vi "GrGFASTAcquireDSO1004.vi"() -> ()   [LabVIEW 2011]
doc: "This example shows how to configure multiple channels and acquire waveforms from multiple channels."
uses:
  <instrlib>/Agilent DSO1000 Series/Public/Data/Read Waveform (Multiple).vi
  <vilib>/Waveform/WDTFileIO.llb/Export Waveforms To Spreadsheet File (1D).vi
  <instrlib>/Agilent DSO1000 Series/Agilent DSO1000 Series.lvlib
panel:
  in  "File Path Control":path=path "E:/Documents/MSU/Research/Measurement/PlateProperties/MulticycleSignal/F100kD4cm.txt"
  in  "stop":bool
  in  "Maximum Time (10000 ms)":u32=10000
  out "Waveform Data":waveform(dbl)[](graph)=[{"t0"=timestamp(-5.9999998484050465e-05 s since 1904-01-01), "dt"=2e-07, "Y"=[0.0, 0.4, 0.0, 0.4, 0.0, 0.4, 0.0, 0.4, 0.4, 0.0, 0.4, 0.0, 0.0, 0.4, 0.4, 0.0, 0.4, 0.0, 0.4, 0.0, 0.0, 0.4, 0.4, 0.0, 0.0, 0.4, 0.0, 0.4, 0.0, 0.4, 0.4, 0.0, 0.0, 0.4, 0.4, 0.0, 0.4, 0.0, 0.0, 0.4, 0.4, 0.0, 0.0, 0.4, 0.4, 0.0, 0.4, 0.0, 0.4, 0.0, 0.0, 0.4, 0.0, 0.4, 0.0, 0.4, 0.0, 0.4, 0.0, 0.4, 0.4, 0.0, 0.0, 0.4, 0.0, 0.4, 0.0, 0.4, 0.0, 0.0, 0.4, 0.0, 0.0, 0.4, 0.0, 0.4, 0.0, 0.4, 0.0, 0.4, 0.0, 0.4, 0.0, 0.4, 0.4, 0.0, 0.0, 0.4, 0.4, 0.0, 0.0, 0.0, 0.0, 0.4, 0.0, 0.4, 0.4, 0.0, 0.0, 0.4, 0.4, 0.0, 0.0, 0.4, 0.0, 0.4, 0.0, 0.4, 0.0, 0.4, 0.0, 0.4, 0.0, 0.4, 0.0, 0.4, 0.0, 0.4, 0.4, 0.0, 0.0, 0.4, 0.4, 0.0, 0.0, 0.4, 0.4, 0.0, 0.0, 0.4, 0.0, 0.4, 0.0, 0.4, 0.4, 0.0, 0.0, 0.4, 0.4, 0.0, 0.0, 0.4, 0.0, 0.4, 0.0, 0.4, 0.0, 0.4, 0.0, 0.4, 0.4, 0.0, 0.4, 0.0, 0.4, 0.0, 0.0, 0.4, 0.0, 0.4, 0.4, 0.0, 0.0, 0.4, 0.0, 0.4, 0.0, 0.4, 0.0, 0.4, 0.0, 0.4, 0.0, 0.4, 0.4, 0.0, 0.4, 0.0, 0.4, 0.0, 0.4, 0.0, 0.4, 0.0, 0.4, 0.0, 0.0, 0.4, 0.0, 0.4, 0.4, 0.0, 0.0, 0.4, 0.4, 0.0, 0.0, 0.4, 0.0, 0.4, 0.0, 0.4, 0.0, 0.4, 0.0, 0.4, 0.0, 0.4, 0.0, 0.4, 0.0, 0.4, 0.0, 0.4, 0.4, 0.0, 0.4, 0.0, 0.0, 0.4, 0.0, 0.4, 0.0, 0.4, 0.0, 0.4, 0.0, 0.4, 0.0, 0.4, 0.0, 0.4, 0.0, 0.4, 0.0, 0.4, 0.0, 0.4, 0.4, 0.0, 0.0, 0.4, 0.4, 0.0, 0.4, 0.0, 0.4, 0.0, 0.4, 0.0, 0.4, 0.0, 0.4, 0.0, 0.0, 0.4, 0.0, 0.4, 0.4, 0.0, 0.0, 0.4, 0.4, 0.4, 0.4, 0.4, 0.4, 0.4, 0.4, 0.0, 0.0, 0.0, 0.0, -0.4, -0.4, 0.0, 0.0, 0.0, 0.0, 0.4, 0.4, 1.2000000000000002, 1.6, 1.2000000000000002, 1.6, 1.6, 1.6, 1.2000000000000002, 0.8, 0.0, -0.4, -1.2000000000000002, -1.6, -2.8000000000000003, -2.8000000000000003, -2.4000000000000004, -2.4000000000000004, -1.2000000000000002, -0.8, 1.2000000000000002, 1.6, 3.6, 3.6, 4.800000000000001, 5.2, 4.4, 4.4, 2.4000000000000004, 2.0, -0.8, -1.2000000000000002, -4.0, -4.4, -6.0, -6.0, -5.6000000000000005, -5.6000000000000005, -2.8000000000000003, -2.4000000000000004, 1.6, 2.0, 5.2, 6.0, 7.2, 7.2, 6.4, 6.0, 3.2, 3.2, -0.8, -1.2000000000000002, -4.4, -4.800000000000001, -6.0, -6.0, -5.2, -5.2, -2.4000000000000004, -2.4000000000000004, 1.2000000000000002, 1.6, 4.0, 4.0, 4.800000000000001, 4.800000000000001, 4.4, 4.4, 2.4000000000000004, 2.0, 0.0, -0.4, -2.0, -2.0, -2.8000000000000003, -2.8000000000000003, -2.0, -2.0, -0.8, -0.8, 0.4, 0.4, 1.6, 1.6, 1.6, 1.6, 1.6, 1.6, 0.8, 0.8, 0.0, 0.0, 0.0, 0.0, -0.4, 0.0, -0.4, 0.0, 0.0, 0.0, 0.0, 0.0, 0.4, 0.4, 0.4, 0.4, 0.4, 0.4, 0.0, 0.4, 0.0, 0.0, 0.4, 0.0, 0.0, 0.0, 0.0, 0.0, 0.0, 0.0, 0.4, 0.0, 0.4, 0.0, 0.4, 0.4, 0.0, 0.0, 0.4, 0.0, 0.4, 0.0, 0.4, 0.0, 0.4, 0.0, 0.4, 0.4, 0.0, 0.4, 0.0, 0.4, 0.0, 0.0, 0.4, 0.0, 0.4, 0.0, 0.4, 0.4, 0.0, 0.0, 0.4, 0.0, 0.4, 0.0, 0.4, 0.0, 0.4, 0.4, 0.0, 0.0, 0.4, 0.4, 0.0, 0.0, 0.4, 0.4, 0.0, 0.0, 0.4, 0.0, 0.4, 0.0, 0.4, 0.0, 0.4, 0.0, 0.4, 0.0, 0.4, 0.4, 0.0, 0.0, 0.4, 0.0, 0.4, 0.0, 0.4, 0.0, 0.4, 0.0, 0.4, 0.4, 0.0, 0.4, 0.0, 0.4, 0.0, 0.4, 0.0, 0.0, 0.4, 0.0, 0.4, 0.0, 0.4, 0.0, 0.4, 0.0, 0.4, 0.0, 0.4, 0.0, 0.4, 0.4, 0.0, 0.0, 0.4, 0.4, 0.0, 0.4, 0.0, 0.0, 0.4, 0.0, 0.0, 0.4, 0.0, 0.4, 0.0, 0.0, 0.4, 0.0, 0.4, 0.0, 0.4, 0.4, 0.0, 0.0, 0.0, 0.0, 0.4, 0.0, 0.4, 0.0, 0.4, 0.4, 0.0, 0.0, 0.4, 0.4, 0.0, 0.4, 0.0, 0.0, 0.4, 0.0, 0.4, 0.4, 0.0, 0.0, 0.0, 0.4, 0.0, 0.0, 0.4, 0.0, 0.4, 0.0, 0.4, 0.0, 0.4, 0.0, 0.4, 0.0, 0.4, 0.0, 0.4, 0.4, 0.0, 0.0, 0.4, 0.0, 0.0, 0.4, 0.0, 0.0, 0.4, 0.4, 0.0, 0.0, 0.0, 0.4, 0.0, 0.0, 0.4, 0.0, 0.4, 0.0, 0.4, 0.0, 0.4, 0.0, 0.4, 0.0, 0.4, 0.0, 0.0, 0.0, 0.4, 0.4, 0.0, 0.0, 0.4, 0.0, 0.4, 0.4, 0.0, 0.0, 0.4]}, {"t0"=timestamp(-5.9999998484050465e-05 s since 1904-01-01), "dt"=2e-07, "Y"=[0.004, 0.0, 0.0, 0.004, 0.0, 0.004, 0.0, 0.004, 0.004, 0.0, 0.004, 0.0, 0.0, 0.004, 0.0, 0.004, 0.0, 0.004, 0.004, 0.0, 0.0, 0.004, 0.004, 0.0, 0.0, 0.004, 0.004, 0.0, 0.004, 0.0, 0.004, 0.0, 0.004, 0.0, 0.0, 0.004, 0.0, 0.004, 0.0, 0.004, 0.0, 0.004, 0.004, 0.0, 0.0, 0.004, 0.0, 0.004, 0.0, 0.004, 0.004, 0.0, 0.0, 0.004, 0.0, 0.004, 0.0, 0.004, 0.0, 0.004, 0.0, 0.004, 0.0, 0.004, 0.0, 0.004, 0.0, 0.004, 0.004, 0.0, 0.004, 0.0, 0.0, 0.004, 0.0, 0.004, 0.0, 0.004, 0.004, 0.0, 0.0, 0.004, 0.0, 0.004, 0.0, 0.004, 0.0, 0.004, 0.0, 0.0, 0.0, 0.004, 0.0, 0.004, 0.004, 0.0, 0.0, 0.004, 0.0, 0.0, 0.0, 0.004, 0.004, 0.0, 0.0, 0.004, 0.0, 0.004, 0.0, 0.004, 0.0, 0.004, 0.0, 0.004, 0.0, 0.004, 0.004, 0.0, 0.004, 0.0, 0.0, 0.004, 0.0, 0.004, 0.0, 0.004, 0.0, 0.0, 0.0, 0.004, 0.004, 0.0, 0.0, 0.004, 0.004, 0.0, 0.0, 0.004, 0.0, 0.004, 0.0, 0.004, 0.004, 0.0, 0.0, 0.004, 0.0, 0.004, 0.0, 0.004, 0.0, 0.004, 0.004, 0.0, 0.0, 0.004, 0.0, 0.004, 0.0, 0.004, 0.0, 0.004, 0.0, 0.004, 0.004, 0.0, 0.0, 0.004, 0.0, 0.004, 0.0, 0.004, 0.004, 0.0, 0.0, 0.004, 0.0, 0.004, 0.0, 0.004, 0.0, 0.004, 0.0, 0.004, 0.0, 0.004, 0.0, 0.004, 0.0, 0.004, 0.0, 0.0, 0.0, 0.004, 0.004, 0.0, 0.004, 0.0, 0.0, 0.004, 0.0, 0.004, 0.0, 0.004, 0.004, 0.0, 0.0, 0.004, 0.004, 0.0, 0.0, 0.004, 0.004, 0.0, 0.0, 0.004, 0.004, 0.0, 0.0, 0.004, 0.0, 0.004, 0.0, 0.004, 0.0, 0.004, 0.004, 0.0, 0.0, 0.0, 0.0, 0.004, 0.0, 0.004, 0.0, 0.004, 0.0, 0.004, 0.004, 0.0, 0.004, 0.0, 0.0, 0.004, 0.004, 0.0, 0.004, 0.0, 0.0, 0.004, 0.0, 0.004, 0.0, 0.004, 0.0, 0.004, 0.0, 0.004, 0.0, 0.004, 0.0, 0.004, 0.004, 0.0, 0.0, 0.004, 0.0, 0.004, 0.004, 0.0, 0.0, 0.004, 0.0, 0.004, 0.0, 0.004, 0.004, 0.0, 0.004, 0.0, 0.0, 0.004, 0.0, 0.004, 0.0, 0.004, 0.0, 0.004, 0.004, 0.0, 0.004, 0.0, 0.004, 0.0, 0.0, 0.004, 0.004, 0.0, 0.0, 0.004, 0.0, 0.004, 0.004, 0.0, 0.004, 0.0, 0.004, 0.0, 0.0, 0.004, 0.0, 0.004, 0.0, 0.004, 0.0, 0.004, 0.0, 0.004, 0.004, 0.0, 0.0, 0.004, 0.0, 0.004, 0.0, 0.004, 0.0, 0.004, 0.004, 0.0, 0.0, 0.004, 0.0, 0.004, 0.0, 0.004, 0.0, 0.004, 0.0, 0.004, 0.0, 0.004, 0.0, 0.004, 0.0, 0.004, 0.004, 0.0, 0.0, 0.004, 0.0, 0.004, 0.0, 0.004, 0.004, 0.0, 0.0, 0.004, 0.0, 0.004, 0.0, 0.004, 0.004, 0.0, 0.0, 0.004, 0.004, 0.0, 0.004, 0.0, 0.004, 0.0, 0.004, 0.0, 0.0, 0.004, 0.0, 0.004, 0.0, 0.004, 0.004, 0.0, 0.0, 0.004, 0.0, 0.004, 0.0, 0.004, 0.004, 0.0, 0.0, 0.004, 0.0, 0.004, 0.004, 0.0, 0.0, 0.004, 0.004, 0.0, 0.0, 0.004, 0.004, 0.0, 0.0, 0.0, 0.0, 0.004, 0.0, 0.004, 0.0, 0.0, 0.0, 0.004, 0.004, 0.0, 0.004, 0.0, 0.0, 0.004, 0.0, 0.004, 0.0, 0.004, 0.004, 0.0, 0.0, 0.004, 0.0, 0.004, 0.0, 0.004, 0.0, 0.004, 0.0, 0.0, 0.0, 0.004, 0.0, 0.004, 0.0, 0.004, 0.004, 0.0, 0.0, 0.004, 0.0, 0.004, 0.004, 0.0, 0.0, 0.0, 0.0, 0.0, 0.0, 0.004, 0.0, 0.004, 0.0, 0.004, 0.0, 0.004, 0.004, 0.0, 0.0, 0.004, 0.0, 0.004, 0.004, 0.0, 0.004, 0.0, 0.0, 0.004, 0.0, 0.004, 0.004, 0.0, 0.004, 0.0, 0.004, 0.0, 0.004, 0.0, 0.0, 0.004, 0.0, 0.004, 0.004, 0.0, 0.0, 0.004, 0.0, 0.004, 0.004, 0.0, 0.0, 0.004, 0.0, 0.0, 0.0, 0.004, 0.0, 0.004, 0.0, 0.004, 0.004, 0.0, 0.004, 0.0, 0.0, 0.004, 0.0, 0.004, 0.004, 0.0, 0.0, 0.004, 0.0, 0.004, 0.004, 0.0, 0.0, 0.0, 0.004, 0.0, 0.0, 0.004, 0.0, 0.004, 0.0, 0.004, 0.0, 0.004, 0.0, 0.0, 0.0, 0.004, 0.0, 0.004, 0.0, 0.004, 0.0, 0.004, 0.004, 0.0, 0.0, 0.004, 0.0, 0.004, 0.0, 0.004, 0.0, 0.004, 0.004, 0.0, 0.004, 0.0, 0.004, 0.0, 0.004, 0.0, 0.0, 0.0, 0.0, 0.004, 0.0, 0.004, 0.0, 0.004, 0.0, 0.004, 0.004, 0.0, 0.004, 0.0, 0.004, 0.0, 0.0, 0.004, 0.0, 0.004, 0.0, 0.004, 0.0, 0.004, 0.0, 0.004, 0.0, 0.004, 0.0, 0.004, 0.0, 0.004, 0.0, 0.004, 0.004, 0.0, 0.0, 0.004]}, {"t0"=timestamp(-5.9999998484050465e-05 s since 1904-01-01), "dt"=2e-07, "Y"=[0.0, 0.0, 0.0, 0.0, 0.0, 0.0, 0.0, 0.0, 0.0, 0.0, 0.0, 0.0, 0.0, 0.0, 0.0, 0.0, 0.0, 0.0, 0.0, 0.0, 0.0, 0.0, 0.0, 0.0, 0.0, 0.0, 0.0, 0.0, 0.0, 0.0, 0.0, 0.0, 0.0, 0.0, 0.0, 0.0, 0.0, 0.0, 0.0, 0.0, 0.0, 0.0, 0.0, 0.0, 0.0, 0.0, 0.0, 0.0, 0.0, 0.0, 0.0, 0.0, 0.0, 0.0, 0.0, 0.0, 0.0, 0.0, 0.0, 0.0, 0.0, 0.0, 0.0, 0.4, 0.0, 0.0, 0.0, 0.0, 0.0, 0.0, 0.0, 0.0, 0.0, 0.0, 0.0, 0.0, 0.0, 0.0, 0.0, 0.4, 0.0, 0.0, 0.0, 0.0, 0.0, 0.0, 0.0, 0.0, 0.0, 0.0, 0.0, 0.0, 0.0, 0.0, 0.0, 0.4, 0.0, 0.0, 0.0, 0.0, 0.0, 0.0, 0.0, 0.0, 0.0, 0.0, 0.0, 0.0, 0.0, 0.0, 0.0, 0.0, 0.0, 0.0, 0.0, 0.0, 0.0, 0.0, 0.0, 0.0, 0.0, 0.0, 0.0, 0.0, 0.0, 0.0, 0.0, 0.0, 0.0, 0.0, 0.0, 0.0, 0.0, 0.0, 0.0, 0.0, 0.0, 0.0, 0.0, 0.0, 0.0, 0.4, 0.0, 0.0, 0.0, 0.0, 0.0, 0.0, 0.0, 0.0, 0.0, 0.0, 0.0, 0.0, 0.0, 0.0, 0.0, 0.0, 0.0, 0.0, 0.0, 0.0, 0.0, 0.0, 0.0, 0.0, 0.0, 0.0, 0.0, 0.0, 0.0, 0.0, 0.0, 0.0, 0.0, 0.0, 0.0, 0.0, 0.0, 0.0, 0.0, 0.0, 0.0, 0.0, 0.0, 0.0, 0.0, 0.0, 0.0, 0.0, 0.0, 0.0, 0.0, 0.0, 0.0, 0.0, 0.0, 0.0, 0.0, 0.0, 0.0, 0.0, 0.0, 0.0, 0.0, 0.0, 0.0, 0.0, 0.0, 0.0, 0.0, 0.0, 0.0, 0.0, 0.0, 0.0, 0.0, 0.0, 0.0, 0.0, 0.0, 0.4, 0.0, 0.0, 0.0, 0.0, 0.0, 0.0, 0.0, 0.0, 0.0, 0.0, 0.0, 0.0, 0.0, 0.0, 0.0, 0.0, 0.0, 0.0, 0.0, 0.0, 0.0, 0.0, 0.0, 0.0, 0.0, 0.0, 0.0, 0.0, 0.0, 0.0, 0.0, 0.0, 0.0, 0.0, 0.0, 0.0, 0.0, 0.0, 0.0, 0.0, 0.0, 0.0, 0.0, 0.0, 0.0, 0.4, 0.0, 0.0, 0.0, 0.0, 0.0, 0.0, 0.0, 0.0, 0.0, 0.0, 0.0, 0.0, 0.0, 0.0, 0.0, 0.0, 0.0, 0.0, 0.0, 0.0, 0.0, 0.0, 0.0, 0.0, 0.0, 0.0, 0.0, 0.0, 0.0, 0.0, 0.0, 0.0, 0.0, 0.0, 0.0, 0.0, 0.0, 0.0, 0.0, 0.0, 0.0, 0.0, 0.0, 0.0, 0.0, 0.0, 0.0, 0.0, 0.0, 0.0, 0.0, 0.0, 0.0, 0.0, 0.0, 0.0, 0.0, 0.0, 0.0, 0.0, 0.0, 0.0, 0.0, 0.0, 0.0, 0.0, 0.0, 0.0, 0.0, 0.0, 0.0, 0.0, 0.0, 0.0, 0.0, 0.0, 0.0, 0.0, 0.0, 0.0, 0.0, 0.4, 0.0, 0.4, 0.0, 0.0, 0.0, 0.0, 0.0, 0.0, 0.0, 0.0, 0.0, 0.0, 0.0, 0.0, 0.0, 0.0, 0.0, 0.0, 0.0, 0.0, 0.0, 0.0, 0.0, 0.0, 0.0, 0.0, 0.0, 0.0, 0.0, 0.0, 0.0, 0.0, 0.0, 0.0, 0.0, 0.0, 0.0, 0.0, 0.0, 0.0, 0.0, 0.0, 0.0, 0.0, 0.0, 0.0, 0.0, 0.0, 0.0, 0.0, 0.0, 0.0, 0.0, 0.0, 0.0, 0.0, 0.0, 0.0, 0.0, 0.0, 0.0, 0.0, 0.0, 0.0, 0.0, 0.0, 0.0, 0.0, 0.0, 0.0, 0.0, 0.0, 0.0, 0.0, 0.0, 0.0, 0.0, 0.0, 0.0, 0.0, 0.0, 0.0, 0.0, 0.0, 0.0, 0.0, 0.0, 0.0, 0.0, 0.0, 0.0, 0.0, 0.0, 0.0, 0.0, 0.0, 0.0, 0.0, 0.0, 0.0, 0.0, 0.0, 0.0, 0.0, 0.0, 0.0, 0.0, 0.0, 0.0, 0.0, 0.0, 0.0, 0.0, 0.0, 0.0, 0.0, 0.0, 0.4, 0.0, 0.0, 0.0, 0.0, 0.0, 0.0, 0.0, 0.0, 0.0, 0.0, 0.0, 0.0, 0.0, 0.0, 0.0, 0.0, 0.4, 0.0, 0.0, 0.0, 0.0, 0.0, 0.0, 0.0, 0.0, 0.0, 0.0, 0.0, 0.0, 0.0, 0.0, 0.0, 0.0, 0.0, 0.0, 0.0, 0.0, 0.0, 0.0, 0.0, 0.0, 0.0, 0.0, 0.0, 0.0, 0.0, 0.0, 0.0, 0.0, 0.0, 0.0, 0.0, 0.0, 0.0, 0.0, 0.0, 0.0, 0.0, 0.0, 0.0, 0.0, 0.0, 0.0, 0.0, 0.0, 0.0, 0.0, 0.0, 0.0, 0.0, 0.0, 0.0, 0.0, 0.0, 0.0, 0.4, 0.0, 0.0, 0.0, 0.0, 0.0, 0.0, 0.0, 0.0, 0.0, 0.0, 0.0, 0.0, 0.0, 0.0, 0.0, 0.0, 0.0, 0.0, 0.0, 0.0, 0.0, 0.0, 0.0, 0.0, 0.0, 0.0, 0.0, 0.0, 0.0, 0.0, 0.0, 0.0, 0.0, 0.0, 0.0, 0.0, 0.0, 0.0, 0.0, 0.0, 0.0, 0.0, 0.0, 0.0, 0.0, 0.0, 0.0, 0.0, 0.0, 0.0, 0.0, 0.0, 0.0, 0.0, 0.0, 0.0]}, {"t0"=timestamp(-5.9999998484050465e-05 s since 1904-01-01), "dt"=2e-07, "Y"=[0.4, 0.0, 0.4, 0.0, 0.0, 0.4, 0.4, 0.0, 0.4, 0.4, 0.4, 0.4, 0.4, 0.4, 0.4, 0.4, 0.4, 0.0, 0.4, 0.0, 0.4, 0.4, 0.0, 0.4, 0.4, 0.0, 0.0, 0.4, 0.4, 0.4, 0.0, 0.4, 0.4, 0.0, 0.4, 0.0, 0.4, 0.0, 0.0, 0.4, 0.4, 0.0, 0.4, 0.0, 0.4, 0.0, 0.0, 0.4, 0.4, 0.0, 0.4, 0.0, 0.4, 0.4, 0.4, 0.0, 0.4, 0.0, 0.0, 0.4, 0.4, 0.0, 0.4, 0.0, 0.4, 0.0, 0.4, 0.0, 0.4, 0.0, 0.0, 0.4, 0.4, 0.0, 0.4, 0.0, 0.4, 0.0, 0.4, 0.0, 0.4, 0.0, 0.4, 0.0, 0.4, 0.0, 0.4, 0.0, 0.4, 0.4, 0.4, 0.0, 0.4, 0.0, 0.4, 0.0, 0.4, 0.4, 0.4, 0.0, 0.4, 0.0, 0.4, 0.0, 0.4, 0.0, 0.4, 0.0, 0.4, 0.0, 0.4, 0.0, 0.4, 0.0, 0.4, 0.4, 0.4, 0.0, 0.4, 0.0, 0.4, 0.0, 0.0, 0.4, 0.4, 0.0, 0.4, 0.0, 0.0, 0.4, 0.4, 0.0, 0.4, 0.0, 0.0, 0.4, 0.4, 0.0, 0.4, 0.4, 0.4, 0.4, 0.4, 0.4, 0.4, 0.0, 0.4, 0.0, 0.4, 0.4, 0.4, 0.0, 0.0, 0.4, 0.4, 0.0, 0.4, 0.4, 0.4, 0.0, 0.4, 0.0, 0.4, 0.0, 0.0, 0.4, 0.0, 0.4, 0.4, 0.0, 0.4, 0.0, 0.4, 0.0, 0.4, 0.0, 0.0, 0.4, 0.4, 0.0, 0.4, 0.0, 0.4, 0.0, 0.0, 0.4, 0.0, 0.4, 0.0, 0.4, 0.0, 0.4, 0.4, 0.0, 0.4, 0.0, 0.4, 0.0, 0.0, 0.4, 0.0, 0.4, 0.0, 0.4, 0.4, 0.0, 0.4, 0.0, 0.4, 0.0, 0.4, 0.0, 0.4, 0.0, 0.4, 0.0, 0.4, 0.0, 0.4, 0.0, 0.0, 0.4, 0.4, 0.0, 0.4, 0.0, 0.4, 0.0, 0.4, 0.0, 0.4, 0.0, 0.4, 0.0, 0.4, 0.0, 0.4, 0.0, 0.0, 0.4, 0.4, 0.0, 0.4, 0.0, 0.4, 0.0, 0.4, 0.0, 0.4, 0.0, 0.4, 0.0, 0.4, 0.4, 0.4, 0.4, 0.0, 0.4, 0.4, 0.0, 0.4, 0.4, 0.4, 0.0, 0.4, 0.0, 0.4, 0.0, 0.4, 0.4, 0.4, 0.4, 0.4, 0.4, 0.4, 0.0, 0.4, 0.4, 0.4, 0.0, 0.4, 0.0, 0.4, 0.0, 0.4, 0.4, 0.4, 0.4, 0.0, 0.4, 0.4, 0.0, 0.0, 0.4, 0.4, 0.0, 0.0, 0.4, 0.4, 0.0, 0.4, 0.0, 0.4, 0.0, 0.0, 0.4, 0.4, 0.0, 0.4, 0.4, 0.4, 0.4, 0.4, 0.0, 0.4, 0.0, 0.4, 0.0, 0.4, 0.0, 0.4, 0.0, 0.4, 0.0, 0.4, 0.0, 0.4, 0.0, 0.0, 0.4, 0.4, 0.0, 0.4, 0.0, 0.4, 0.4, 0.4, 0.0, 0.4, 0.0, 0.4, 0.0, 0.4, 0.0, 0.4, 0.0, 0.4, 0.0, 0.4, 0.4, 0.4, 0.4, 0.4, 0.0, 0.4, 0.0, 0.4, 0.0, 0.4, 0.0, 0.0, 0.4, 0.4, 0.0, 0.4, 0.0, 0.4, 0.0, 0.4, 0.0, 0.4, 0.4, 0.0, 0.4, 0.4, 0.4, 0.4, 0.0, 0.4, 0.0, 0.4, 0.0, 0.4, 0.0, 0.4, 0.0, 0.4, 0.0, 0.0, 0.4, 0.4, 0.0, 0.4, 0.0, 0.4, 0.0, 0.0, 0.4, 0.0, 0.4, 0.0, 0.4, 0.4, 0.0, 0.4, 0.0, 0.4, 0.0, 0.0, 0.4, 0.4, 0.4, 0.4, 0.0, 0.4, 0.0, 0.4, 0.0, 0.0, 0.4, 0.4, 0.0, 0.0, 0.4, 0.4, 0.0, 0.4, 0.4, 0.4, 0.0, 0.0, 0.4, 0.4, 0.0, 0.0, 0.4, 0.4, 0.0, 0.0, 0.4, 0.4, 0.0, 0.0, 0.4, 0.4, 0.0, 0.4, 0.0, 0.0, 0.4, 0.4, 0.0, 0.4, 0.0, 0.4, 0.4, 0.4, 0.4, 0.4, 0.0, 0.0, 0.4, 0.4, 0.0, 0.0, 0.4, 0.4, 0.4, 0.4, 0.0, 0.0, 0.4, 0.4, 0.0, 0.4, 0.0, 0.4, 0.0, 0.0, 0.4, 0.4, 0.0, 0.4, 0.0, 0.4, 0.0, 0.4, 0.0, 0.4, 0.0, 0.0, 0.4, 0.4, 0.4, 0.4, 0.4, 0.4, 0.0, 0.4, 0.0, 0.4, 0.0, 0.4, 0.4, 0.4, 0.4, 0.4, 0.0, 0.4, 0.0, 0.4, 0.4, 0.0, 0.4, 0.0, 0.4, 0.4, 0.0, 0.4, 0.4, 0.4, 0.0, 0.4, 0.4, 0.4, 0.0, 0.0, 0.4, 0.4, 0.0, 0.4, 0.0, 0.4, 0.0, 0.0, 0.4, 0.4, 0.0, 0.4, 0.0, 0.4, 0.4, 0.4, 0.0, 0.4, 0.0, 0.4, 0.0, 0.4, 0.0, 0.4, 0.4, 0.4, 0.0, 0.4, 0.0, 0.4, 0.4, 0.4, 0.0, 0.4, 0.0, 0.4, 0.0, 0.0, 0.4, 0.4, 0.4, 0.4, 0.4, 0.4, 0.0, 0.4, 0.0, 0.4, 0.0, 0.4, 0.0, 0.4, 0.0, 0.4, 0.4, 0.4, 0.0, 0.4, 0.0, 0.4, 0.0, 0.4, 0.4, 0.0, 0.4, 0.4, 0.0, 0.4, 0.0, 0.4, 0.0, 0.4, 0.0]}]
  in  "VISA resource name":refnum<visa-resource-name>
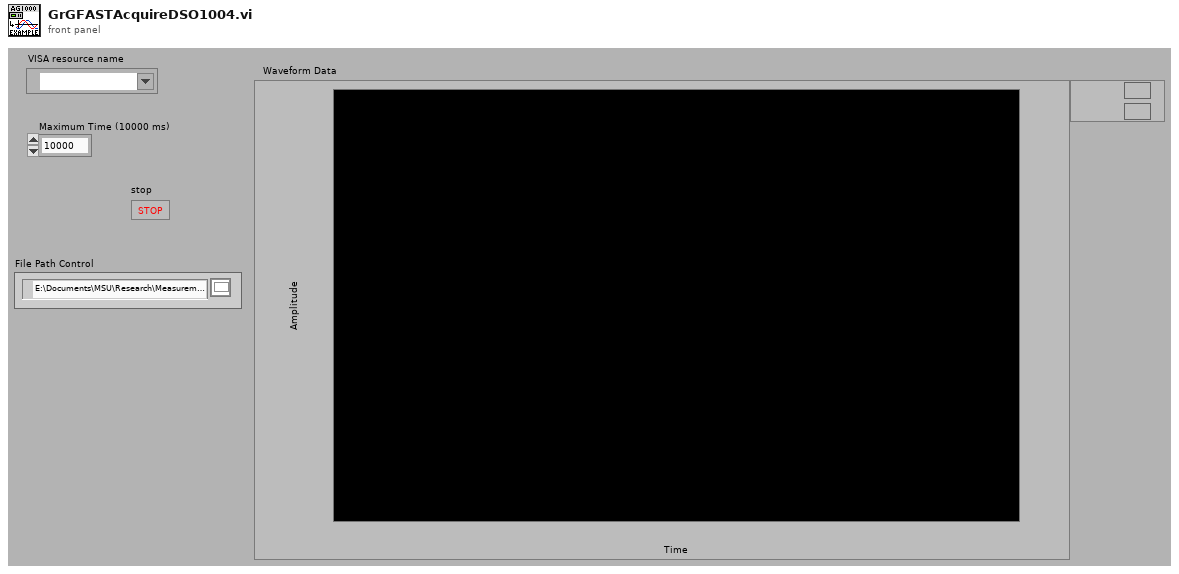
[diagram p1: front panel]
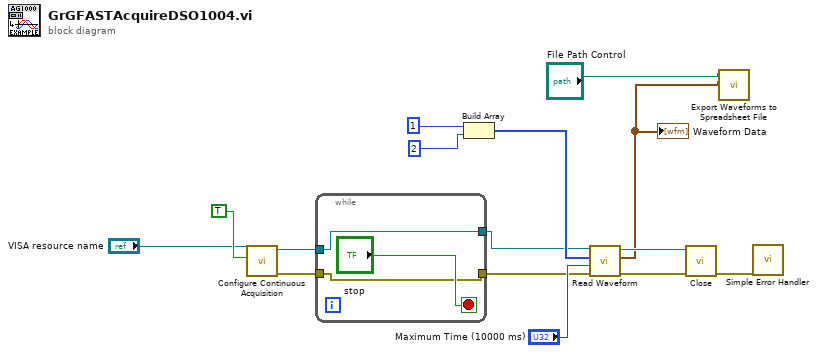
[diagram p0: block diagram]
diagram:
  n1 = call <instrlib>:"Configure Continuous Acquisition.vi"("Enable Continuous Acquisition (T:Enable)"=TRUE, "VISA resource name"="VISA resource name") -> ("error out"=w6:errorcluster, "VISA resource name out"=w4:refnum<visa-resource-name>)  [unwired: 8 in]
  n2 = while {
    tunnel: w6 -> [w17]
    tunnel: [w17] -> w5
    tunnel: w4 -> [w16]
    tunnel: [w16] -> w3
    stop <- "stop" stop-if-true
  }
  n3 = Build Array(u32 1 ("milliseconds to wait"), u32 2 ("milliseconds to wait")) -> (w9:u32[])
  n4 = call-poly <instrlib>:"Read Waveform.vi"("error in (no error)"=w5, "Maximum Time (10000 ms)"="Maximum Time (10000 ms)", "Channels"=w9, "VISA resource name"=w3) -> ("error out"=w14:errorcluster, "Waveform Data"=w1:waveform(dbl)[], "VISA resource name out"=w12:refnum<visa-resource-name>)  [unwired: 5 in]
  "Waveform Data" <- w1
  n5 = call <instrlib>:"Close.vi"("error in (no error)"=w14, "VISA resource name"=w12) -> ("error out"=w13:errorcluster)  [unwired: 9 in]
  n6 = call-poly <vilib>:"Export Waveforms to Spreadsheet File.vi"("waveforms"=w1, "file path (dialog if empty)"="File Path Control") -> ()  [unwired: 8 in, 2 out]
  n7 = call <vilib>:"Simple Error Handler.vi"("error in (no error)"=w13) -> ()  [unwired: 4 in, 5 out]
